vi "Window Size Changed.vi"(8 "error in":errorcluster, 9 "Module Name":string, 10 "窗口边界":T1, 11 "Module ID":i32=-1) -> (0 "error out":errorcluster)   [LabVIEW 2018, in "ModuleInterface.lvlib"]
doc: "广播窗口的新尺寸\n_____\nCreated using DQMH Event Scripter 7.0.1.1316."
uses:
  ModuleInterface.lvlib
  <vilib>/Utility/miscctls.llb/LVRectTypeDef.ctl
  Window Size Changed Argument--cluster.ctl
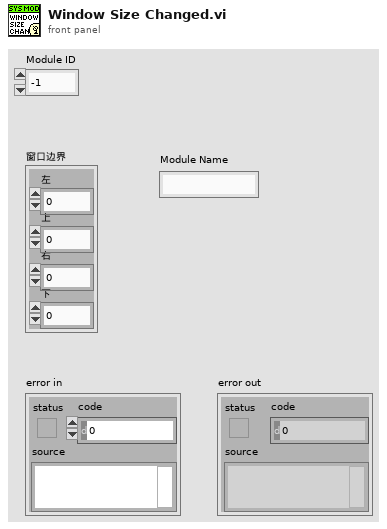
[diagram p1: front panel]
types:
  T1 = typedef "LVRectTypeDef.ctl" = cluster{"Left":i16, "Top":i16, "Right":i16, "Bottom":i16}
  T2 = typedef "ModuleInterface.lvlib/Window Size Changed Argument--cluster.ctl" = cluster{"Module ID":i32, "Module Name":string, "窗口边界":T1}
  T3 = typedef "ModuleInterface.lvlib/Broadcast Events--cluster.ctl" = cluster{"Module Did Init":refnum<user-event>, "Status Updated":refnum<user-event>, "Error Reported":refnum<user-event>, "Module Did Stop":refnum<user-event>, "Update Module Execution Status":refnum<user-event>, "Function Selected":refnum<user-event>, "Window Size Changed":refnum<user-event>}
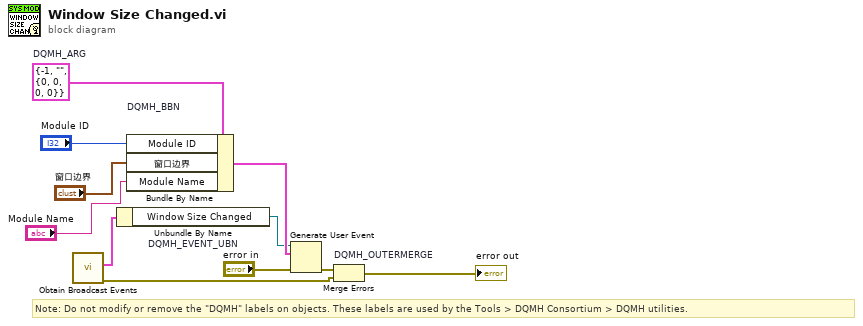
[diagram p0: block diagram]
diagram:
  w6 = T2 {"Module ID"=-1, "Module Name"="", "窗口边界"={"Left"=0, "Top"=0, "Right"=0, "Bottom"=0}}  # DQMH_ARG
  # "Note: Do not modify or remove the \"DQMH\" labels on objects. These labels are used by the Tools > DQMH Consortium > DQMH utilities."
  n1 = call "Obtain Broadcast Events.vi"() -> ("error out"=w3:errorcluster, "ModuleInterface Broadcast Events"=w2:T3)  [unwired: 10 in]
  n2 = Unbundle By Name "DQMH_EVENT_UBN"(w2) -> ("Window Size Changed"=w8:refnum<user-event>)
  n3 = Bundle By Name "DQMH_BBN"(cluster=w6, "Module ID"="Module ID", "窗口边界"="窗口边界", "Module Name"="Module Name") -> (w9:T2)
  n4 = Generate User Event(user event=w8, event data cluster=w9, error in="error in") -> (error out=w7:errorcluster)  [unwired: 1 in, 1 out]
  n5 = Merge Errors "DQMH_OUTERMERGE"(w7, w3) -> (→"error out":errorcluster)
